vi "LED Matrix Image.vi"(4 "Brightness":u8=50 max=100 step=1, 6 "Factor":dbl=2.5, 8 "error in (no error)":errorcluster, 9 "image depth":i32, 10 "image":u8[](array[numeric]), 11 "Refnum in":refnum<k20>) -> (0 "error out":errorcluster, 3 "Refnum out":refnum<k20>, 5 "LED Matrix":picture)   [LabVIEW 2013]
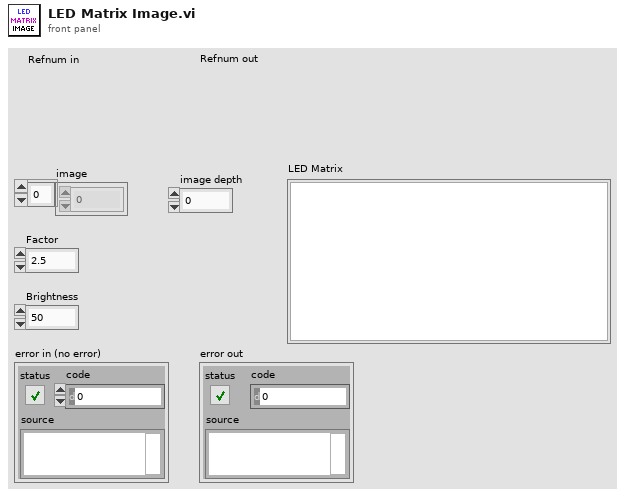
[diagram p1: front panel]
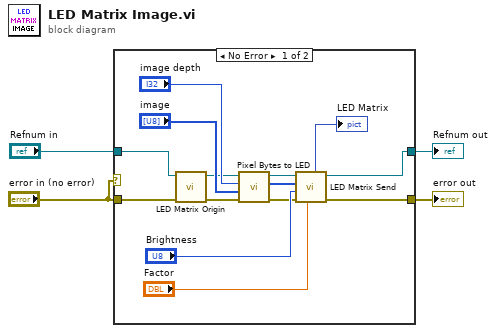
[diagram p0: block diagram]
diagram:
  n1 = case shown="No Error" "error in (no error)" {
    tunnel: "error in (no error)" -> [w8 w19]
    tunnel: "Refnum in" -> [w7 w20]
    tunnel: [w6 w19] -> w3
    tunnel: [w5 w20] -> w4
    frame No Error {
      n2 = call "LED Matrix Origin.vi"("error in (no error)"=w8, "Refnum in"=w7) -> ("error out"=w17:errorcluster, "Refnum out"=w15:refnum<k20>)  [unwired: 8 in]
      n3 = call "Pixel Bytes to LED.vi"("error in (no error)"=w17, "image"="image", "image depth"="image depth", "Refnum in"=w15) -> ("error out"=w11:errorcluster, "LED Data Out"=w13:u32[], "Refnum out"=w12:refnum<k20>)  [unwired: 5 in]
      n4 = call "LED Matrix Send.vi"("Gamma"="Factor", "error in (no error)"=w11, "Brightness"="Brightness", "Data"=w13, "Refnum in"=w12) -> ("error out"=w6:errorcluster, "Refnum out"=w5:refnum<k20>, "LED Matrix"=→"LED Matrix":picture)  [unwired: 3 in]
    }
    frame Error {
    }
  }
  "Refnum out" <- w4
  "error out" <- w3
